vi "Delacor_lib_QMH_Process Error Variant.vi"(8 "error in":errorcluster, 11 "Message Data":variant) -> (0 "error out":errorcluster, 1 "Error Debug":string, 2 "Error":errorcluster)   [LabVIEW 2024, in "RQMHMessageQueue.lvclass"]
doc: "____\nDQMH Framework: Palette 7.1.0.1503\nCopyright (c) 2025, DQMH Consortium"
uses:
  RQMHMessageQueue.lvclass
  <vilib>/Utility/error.llb/Error Cluster From Error Code.vi
  <vilib>/ErrorRing/Error Ring.xnode
  RQMHMessageQueue.lvclass/RQMHMessageQueue.ctl
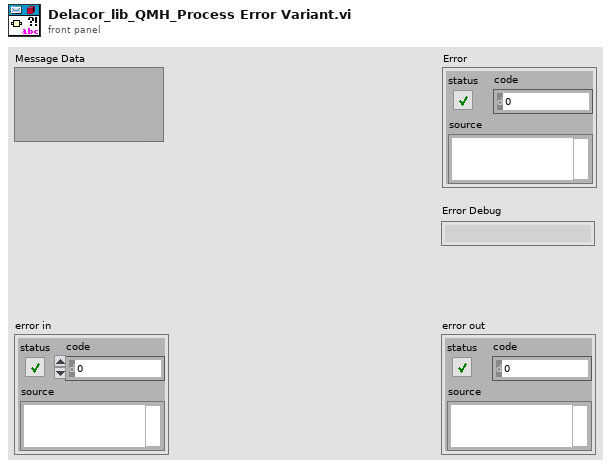
[diagram p1: front panel]
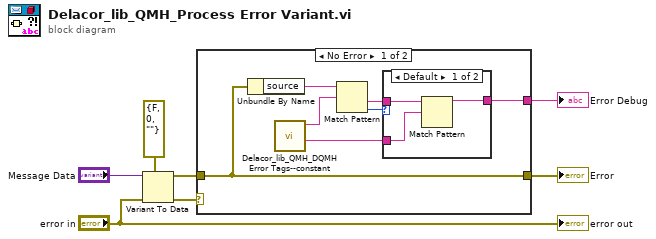
[diagram p0: block diagram]
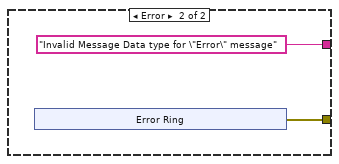
[diagram p3: hidden frame]
diagram:
  n1 = Variant To Data(error in="error in", type=errorcluster {"status"=FALSE, "code"=0, "source"=""} ("error constant"), Variant="Message Data") -> (data=w5:errorcluster, error out=w2:errorcluster)
  n2 = case shown="No Error" w2 {
    tunnel: w5 -> [w8 _]
    tunnel: [w9 "Invalid Message Data type for \"Error\" message" ("source")] -> w4
    tunnel: [w8 w18] -> w1
    frame No Error {
      n3 = Unbundle By Name(w8) -> ("source"=w14:string)
      n4 = call "Delacor_lib_QMH_DQMH Error Tags--constant.vi"() -> ("Close Tag"=w10:string, "Open Tag"=w13:string)  [unwired: 10 in]
      n5 = Match Pattern(string=w14, regular expression=w13) -> (after substring=w11:string, offset past match=w12:i32)  [unwired: 1 in, 2 out]
      n6 = case shown="Default" w12 {
        tunnel: w11 -> [w17 _]
        tunnel: w10 -> [w16 _]
        tunnel: [w15 _] -> w9
        frame Default {
          n7 = Match Pattern(string=w17, regular expression=w16) -> (before substring=w15:string)  [unwired: 1 in, 3 out]
        }
        frame -1 {
        }
      }
    }
    frame Error {
      n8 = xnode "Error Ring"() -> ("error out"=w18:errorcluster)
    }
  }
  "Error" <- w1
  "Error Debug" <- w4
  "error out" <- "error in"
